vi "GetAttributeViString.vi"(7 "AttributeValueBufferSize":i32=256 caption="AttributeValueBufferSize (256)", 8 "error in (no error)":errorcluster {"code" format="%.0x"}, 9 "AttributeID":u32(ring)=1250201 items=["ACTIVE_MARKER"=1250201, "CATALOG_CURRENT_MEASUREMENT_NAME"=1150676, "CATALOG_CURRENT_PERSONALITY_NAME"=1150677, "DISPLAY_TEXT"=1150119, "DRIVER_SETUP"=1050007, "INPUT_RF_CORRECTION_COMMENT"=1150737, "INPUT_RF_CORRECTION_DESCRIPTION"=1150738, "INSTRUMENT_FIRMWARE_REVISION"=1050510, "INSTRUMENT_MANUFACTURER"=1050511, "INSTRUMENT_MODEL"=1050512, "IO_RESOURCE_DESCRIPTOR"=1050304], 10 "RepCapIdentifier":string, 11 "instrument handle":refnum<k15>) -> (0 "error out":errorcluster {"code" format="%.0x"}, 2 "AttributeValue":string, 3 "instrument handle out":refnum<k15>)   [LabVIEW 2009, in "Keysight XSAn.lvlib"]
doc: "Gets a String attribute from the instrument driver.\nThe following Attributes are supported:\n\nACTIVE_MARKER\nCATALOG_CURRENT_MEASUREMENT_NAME\nCATALOG_CURRENT_PERSONALITY_NAME\nDISPLAY_TEXT\nDRIVER_SETUP\nGROUP_CAPABILITIES\nINPUT_RF_CORRECTION_COMMENT\nINPUT_RF_CORRECTION_DESCRIPTION\nINSTRUMENT_FIRMWARE_REVISION\nINSTRUMENT_MANUFACTURER\nINSTRUMENT_MODEL\nIO_RESOURCE_DESCRIPTOR"
uses:
  <instrlib>/Keysight XSAn/Keysight XSAn.lvlib
  AgXSAn.dll
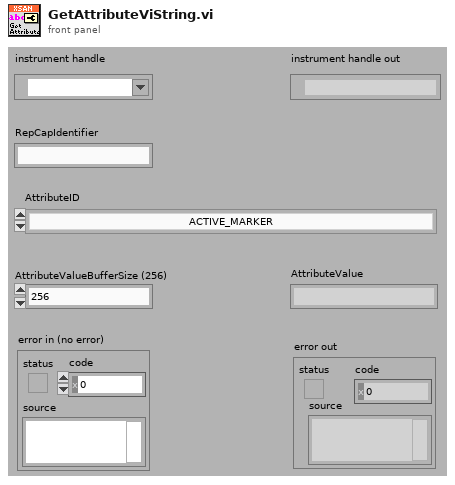
[diagram p1: front panel]
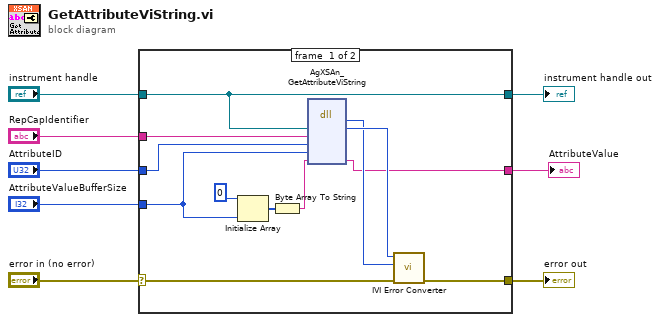
[diagram p0: block diagram]
diagram:
  n1 = case shown="No Error" "error in (no error)" {
    selector: "error in (no error)" -> [w18 w22]
    tunnel: [w17 w22] -> w8
    tunnel: "instrument handle" -> [w10 w21]
    tunnel: "RepCapIdentifier" -> [w16 _]
    tunnel: "AttributeID" -> [w15 _]
    tunnel: "AttributeValueBufferSize" -> [w9 _]
    tunnel: [w11 _] -> w2
    tunnel: [w10 w21] -> w1
    frame #0 {
      n2 = Initialize Array(u8 0 ("element"), w9) -> (w13:u8[])
      n3 = Byte Array To String(unsigned byte array=w13) -> (string=w14:string)
      n4 = dll-call lib="AgXSAn**.dll" fn="AgXSAn_GetAttributeViString"("Vi"=w10, "RepCapIdentifier"=w16, "AttributeID"=w15, "AttributeValueBufferSize"=w9, "AttributeValue"=w14) -> ("return type"=w19:i32, "Vi"=w20:u32, "AttributeValue"=w11:string)  [unwired: 6 in, 2 out]
      n5 = call <instrlib>:"IVI Error Converter.vi"("error in (no error)"=w18, "IVI error code (0)"=w19, "instrument handle"=w20) -> ("error out"=w17:errorcluster)  [unwired: 7 in, 1 out]
    }
    frame #1 {
    }
  }
  "error out" <- w8
  "instrument handle out" <- w1
  "AttributeValue" <- w2
